vi "Sizeof.Scalar.vi"(11 "data type":T1) -> (2 "bitshift count":u8, 3 "size in bytes":i32)   [LabVIEW 2016, in "VeriStand Data.lvlib"]
doc: "Provides the size in bytes of the specified <B>data type</B>."
uses:
  VeriStand Data.lvlib
  Typedefs/Typedefs.Data Types.ctl
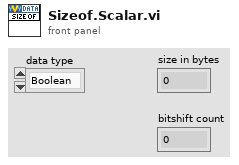
[diagram p1: front panel]
types:
  T1 = typedef "VeriStand Data.lvlib/Typedefs.Data Types.ctl" = enum16{"Boolean", "Single", "Double", "I8", "I16", "I32", "I64", "U8", "U16", "U32", "U64"}
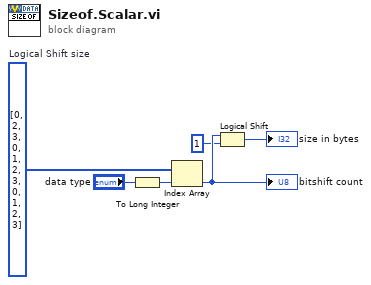
[diagram p0: block diagram]
diagram:
  w5 = u8[] [0, 2, 3, 0, 1, 2, 3, 0, 1, 2, 3]  # Logical Shift size
  n1 = To Long Integer(number="data type") -> (32bit integer=w4:i32)
  n2 = Index Array(array=w5, index=w4) -> (element=w3:u8)
  "bitshift count" <- w3
  n3 = Logical Shift(y=w3, x=1) -> (x << y=→"size in bytes":i32)
